vi "Page_Dialog_Quit.vi"(6 "dialog info":T1, 8 "error in (no error)":errorcluster, 9 "data":variant, 10 "Target":refnum<vi>, 11 "Class in":refnum<class "IB_MSI.lvclass">) -> (0 "error out":errorcluster, 3 "Class out":refnum<class "IB_MSI.lvclass">)   [LabVIEW 2020, in "IB_MSI.lvclass"]
uses:
  <vilib>/AppBuilder/IB_Classes/MSI/IB_MSI.lvclass
  <vilib>/AppBuilder/IB_Classes/MSI/IB_MSI.lvclass/IB_MSI.ctl
  <vilib>/AppBuilder/IB_Classes/Installer/Installer.lvclass
  <resource>/Framework/Providers/Builds/Installer/CDK_sTypeDef_Languages.ctl
  <resource>/Framework/Providers/Builds/Installer/Pages/controls/IB_UI_Page_Dialog_Info_References.ctl
  <resource>/Framework/Providers/Common/provcom_BrowseProjectFile2.ctl
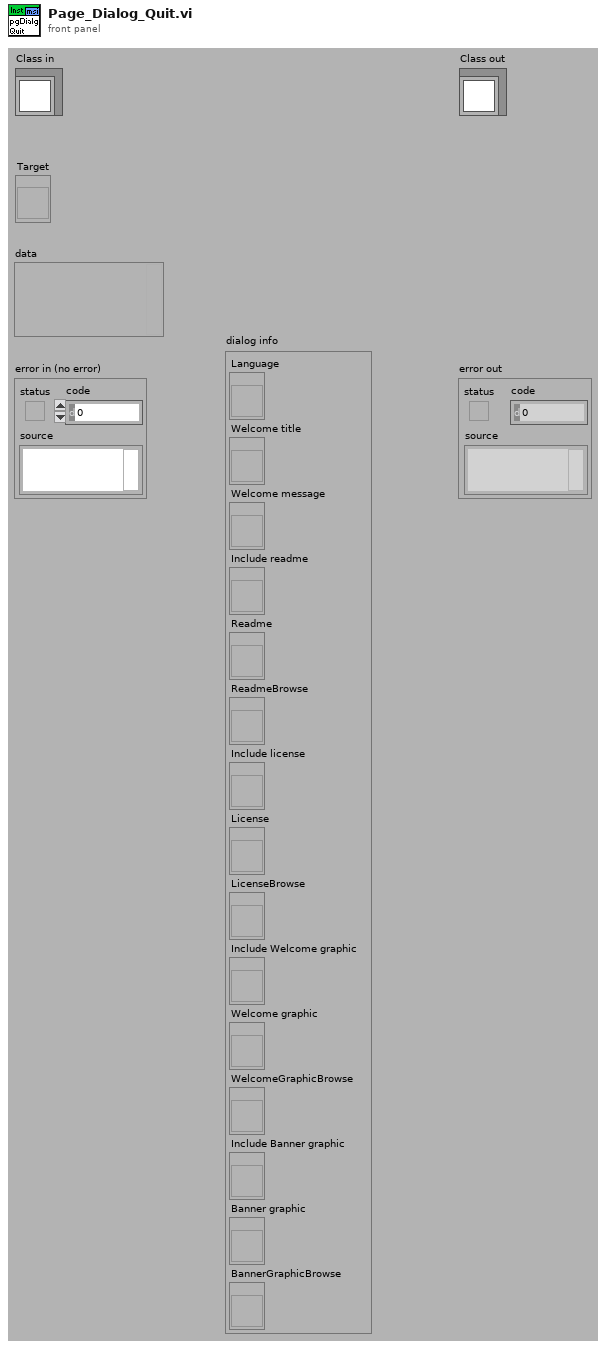
[diagram p1: front panel]
types:
  T1 = typedef "IB_UI_Page_Dialog_Info_References.ctl" = cluster{"Language":refnum<vi>, "Welcome title":refnum<vi>, "Welcome message":refnum<vi>, "Include readme":refnum<vi>, "Readme":refnum<vi>, "ReadmeBrowse":refnum<vi>, "Include license":refnum<vi>, "License":refnum<vi>, "LicenseBrowse":refnum<vi>, "Include Welcome graphic":refnum<vi>, "Welcome graphic":refnum<vi>, "WelcomeGraphicBrowse":refnum<vi>, "Include Banner graphic":refnum<vi>, "Banner graphic":refnum<vi>, "BannerGraphicBrowse":refnum<vi>}
  T2 = typedef "IB_MSI.ctl" = cluster{"upgradeCode":string, "distID":string, "windowMessage":string, "windowTitle":string, "arpPhone":string, "arpContact":string, "arpURL":string, "arpCompany":string, "licenseID":string, "licensePath":path, "welcomeImageID":string, "welcomeImagePath":path, "bannerImageID":string, "bannerImagePath":path, "osCheck":i32, "msiFileName":string, "cabFileName":string, "hwOption":T3, "hwPath":path, "regGroup":refnum<class "IB_RegGroup.lvclass">[], "regDest":refnum<class "IB_RegDest.lvclass">[], "selectedDists":refnum<class "IB_DistPart.lvclass">[], "installedDists":refnum<class "IB_DistPart.lvclass">[], "postInstallSteps":refnum<class "IB_Post_Install_Step.lvclass">[], "preUninstallSteps":refnum<class "IB_Post_Install_Step.lvclass">[], "winsec.certificate":string, "winsec.timestamp":string, "winsec.description":string, "autoselect drivers":bool, "hide non-runtimes":bool}
  T3 = typedef "CDK_sTypeDef_HWImportOption.ctl" = enum16{"<none>", "Merge", "Replace", "Dialog"}
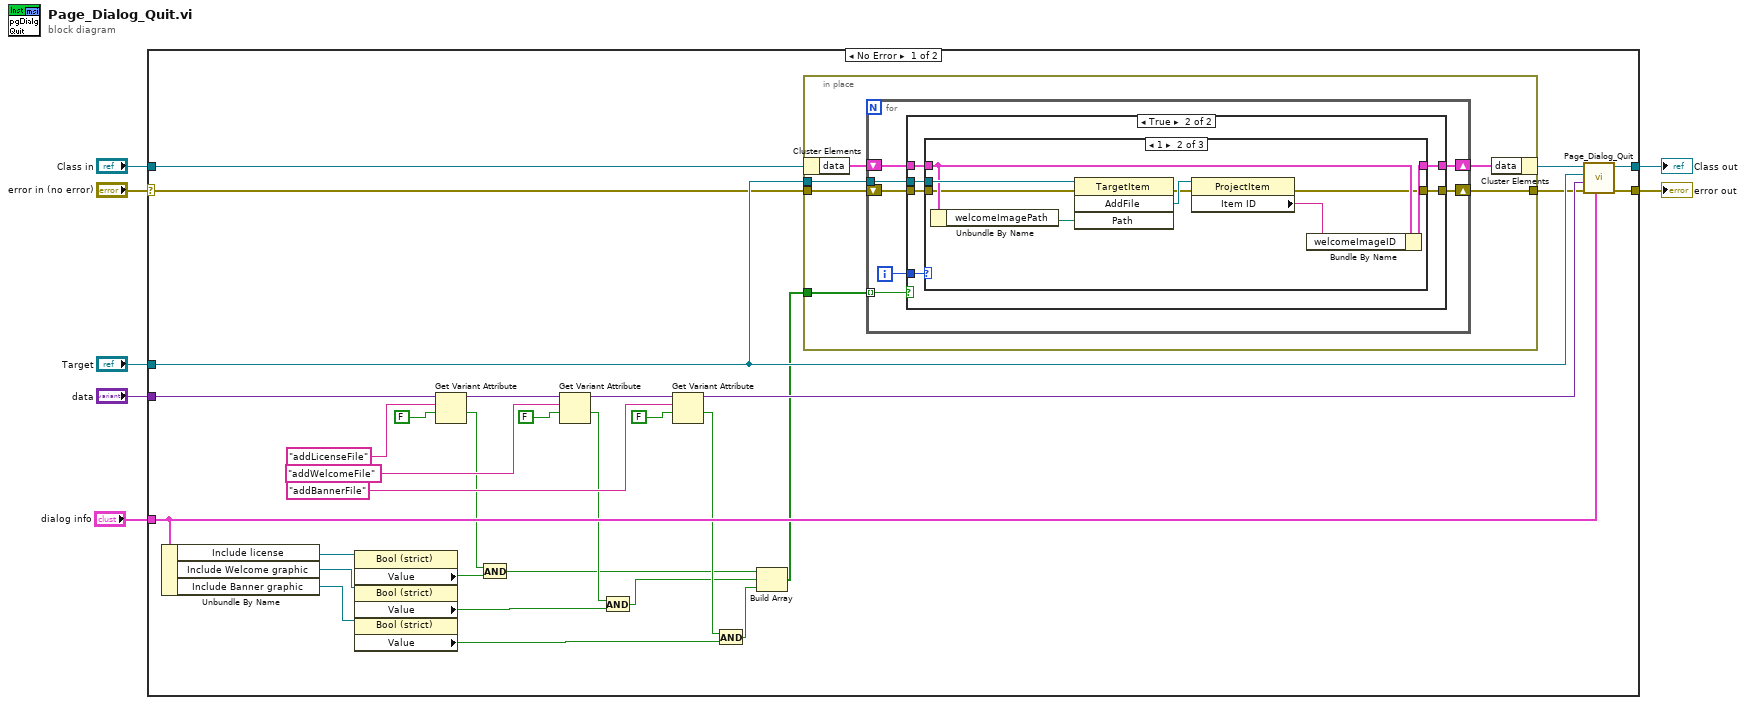
[diagram p0: block diagram]
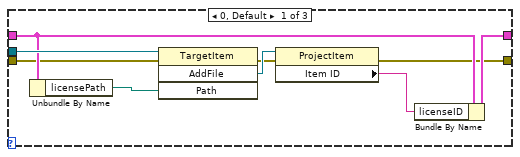
[diagram p3: hidden frame]
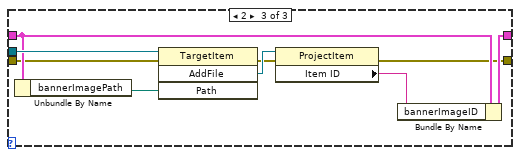
[diagram p4: hidden frame]
diagram:
  n1 = case shown="No Error" "error in (no error)" {
    selector: "error in (no error)" -> [w9 w88]
    tunnel: [w38 w88] -> w7
    tunnel: [w37 w87] -> w6
    tunnel: "dialog info" -> [w36 _]
    tunnel: "data" -> [w24 _]
    tunnel: "Target" -> [w14 _]
    tunnel: "Class in" -> [w16 w87]
    frame No Error {
      n2 = Unbundle By Name(w36) -> ("Include license"=w35:refnum<vi>, "Include Welcome graphic"=w34:refnum<vi>, "Include Banner graphic"=w33:refnum<vi>)
      n3 = property class="Bool (strict)"(reference=w35) -> ("Value"=w21:bool)  [unwired: 1 in, 2 out]
      n4 = property class="Bool (strict)"(reference=w34) -> ("Value"=w19:bool)  [unwired: 1 in, 2 out]
      n5 = property class="Bool (strict)"(reference=w33) -> ("Value"=w18:bool)  [unwired: 1 in, 2 out]
      n6 = Get Variant Attribute(Variant=w24, name="addLicenseFile", default value (empty Variant)=FALSE) -> (duplicate Variant=w29:variant, value=w22:bool)  [unwired: 1 in, 2 out]
      n7 = And(x=w22, y=w21) -> (x .and. y?=w13:bool)
      n8 = Get Variant Attribute(Variant=w29, name="addWelcomeFile", default value (empty Variant)=FALSE) -> (duplicate Variant=w32:variant, value=w20:bool)  [unwired: 1 in, 2 out]
      n9 = And(x=w20, y=w19) -> (x .and. y?=w12:bool)
      n10 = Get Variant Attribute(Variant=w32, name="addBannerFile", default value (empty Variant)=FALSE) -> (duplicate Variant=w23:variant, value=w17:bool)  [unwired: 1 in, 2 out]
      n11 = And(x=w17, y=w18) -> (x .and. y?=w11:bool)
      n12 = Build Array(w13, w12, w11) -> (w10:bool[])
      n13 = in-place {
        in-place-border: w14 -> [w44]
        in-place-border: w10 -> [w41]
        in-place-border: w9 -> [w40]
        in-place-border: [w39] -> w8
        n14 = in-place-cluster #1(w16) -> ("data"=w43:T2)
        n15 = for {
          tunnel: w44 -> [w51]
          tunnel: w41 -> [w48] mode=indexing
          shift-right: [w49] -> w42
          shift-left: w43 -> [w50]
          shift-right: [w45] -> w39
          shift-left: w40 -> [w46]
          i -> [w47]
          n16 = case shown="True" w48 {
            tunnel: w51 -> [_ w59]
            tunnel: w50 -> [w53 w58]
            tunnel: [w53 w57] -> w49
            tunnel: w47 -> [_ w56]
            tunnel: w46 -> [w52 w55]
            tunnel: [w52 w54] -> w45
            frame False {
            }
            frame True {
              n17 = case shown="1" w56 {
                tunnel: w59 -> [w67 w76 w85]
                tunnel: w58 -> [w65 w74 w83]
                tunnel: [w63 w72 w81] -> w57
                tunnel: w55 -> [w62 w71 w78]
                tunnel: [w60 w69 w80] -> w54
                frame 0, Default {
                  n18 = Unbundle By Name(w65) -> ("licensePath"=w66:path)
                  n19 = invoke class="TargetItem" method="AddFile"(reference=w67, error in=w62, "Path"=w66) -> (error out=w61:errorcluster, "AddFile"=w68:refnum<vi>)  [unwired: 1 in, 2 out]
                  n20 = property class="ProjectItem"(reference=w68, error in=w61) -> (error out=w60:errorcluster, "Item ID"=w64:string)  [unwired: 1 out]
                  n21 = Bundle By Name(cluster=w65, "licenseID"=w64) -> (w63:T2)
                }
                frame 1 {
                  n22 = Unbundle By Name(w74) -> ("welcomeImagePath"=w75:path)
                  n23 = invoke class="TargetItem" method="AddFile"(reference=w76, error in=w71, "Path"=w75) -> (error out=w70:errorcluster, "AddFile"=w77:refnum<vi>)  [unwired: 1 in, 2 out]
                  n24 = property class="ProjectItem"(reference=w77, error in=w70) -> (error out=w69:errorcluster, "Item ID"=w73:string)  [unwired: 1 out]
                  n25 = Bundle By Name(cluster=w74, "welcomeImageID"=w73) -> (w72:T2)
                }
                frame 2 {
                  n26 = Unbundle By Name(w83) -> ("bannerImagePath"=w84:path)
                  n27 = invoke class="TargetItem" method="AddFile"(reference=w85, error in=w78, "Path"=w84) -> (error out=w79:errorcluster, "AddFile"=w86:refnum<vi>)  [unwired: 1 in, 2 out]
                  n28 = property class="ProjectItem"(reference=w86, error in=w79) -> (error out=w80:errorcluster, "Item ID"=w82:string)  [unwired: 1 out]
                  n29 = Bundle By Name(cluster=w83, "bannerImageID"=w82) -> (w81:T2)
                }
              }
            }
          }
        }
        n30 = in-place-cluster #1("data"=w42) -> (w15:refnum<class "IB_MSI.lvclass">)
      }
      n31 = call-parent "Page_Dialog_Quit.vi"("dialog info"=w36, "error in (no error)"=w8, "data"=w23, "Target"=w14, "Class in"=w15) -> ("error out"=w38:errorcluster, "Class out"=w37:refnum<class "IB_MSI.lvclass">)  [unwired: 5 out]
    }
    frame Error {
    }
  }
  "error out" <- w7
  "Class out" <- w6
